vi "Main.vi"(8 "error in (no error)":errorcluster, 11 "App in":refnum<class "App.lvclass">) -> (0 "error out":errorcluster)   [LabVIEW 2020, in "Volatus.lvlib"]
uses:
  Volatus.lvlib
  App/App.lvclass
  VolatusCoreTask/VolatusCoreTask.lvclass
  C:/Program Files (x86)/National Instruments/LabVIEW 2020/vi.lib/ActorFramework/Actor/Actor.lvclass
  <vilib>/ActorFramework/Actor/Actor.lvclass
  lv-promises/Promises/Promise/Promise.lvclass
  lv-promises/Promises/Error Result/Error Result.lvclass
  lv-promises/Promises/Future/Future.lvclass
  C:/dev/lv20CE/relink/lv-promises/Promises/Value/Value.lvclass
  C:/dev/lv20CE/relink/lv-promises/Promises/Error Result/Error Result.lvclass
  C:/dev/lv20CE/relink/lv-volatus/Volatus/Task/Task.lvclass
  C:/dev/lv20CE/relink/lv-volatus/Volatus/APIRegistrationHandler/APIRegistrationHandler.lvclass
  C:/dev/lv20CE/relink/lv-volatus/Volatus/TaskStateHandler/TaskStateHandler.lvclass
  C:/dev/lv20CE/relink/lv-volatus/Volatus/VectoMessageHandler/VectoMessageHandler.lvclass
  C:/dev/lv20CE/relink/lv-volatus/Volatus/VolatusCoreTask/VolatusCoreTask.lvclass
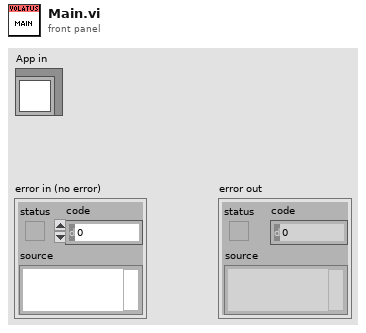
[diagram p1: front panel]
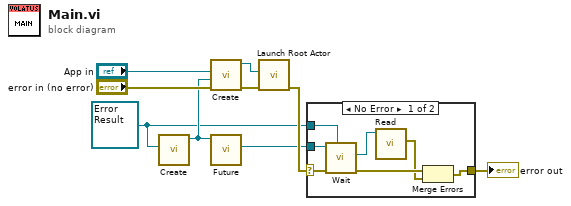
[diagram p0: block diagram]
diagram:
  w2 = refnum<class "Error Result.lvclass"> refnum ("Futures:Error Result.lvclass")
  n1 = call "Create.vi"("Result Type"=w2) -> ("Promise"=w4:refnum<class "Promise.lvclass">)  [unwired: 9 in, 1 out]
  n2 = call "Create.vi"("error in (no error)"="error in (no error)", "Promise"=w4, "App"="App in") -> ("error out"=w6:errorcluster, "VolatusCore out"=w5:refnum<class "VolatusCoreTask.lvclass">)  [unwired: 7 in]
  n3 = call "Future.vi"("Promise in"=w4) -> ("Future"=w3:refnum<class "Future.lvclass">)  [unwired: 9 in, 1 out]
  n4 = call <vilib>:"Launch Root Actor.vi"("error in (no error)"=w6, "Actor"=w5) -> ("error out"=w9:errorcluster)  [unwired: 8 in, 1 out]
  n5 = case shown="No Error" w9 {
    selector: w9 -> [w15 w17]
    tunnel: w3 -> [w16 _]
    tunnel: w2 -> [w14 _]
    tunnel: [w10 w17] -> w1
    frame No Error {
      n6 = call "Wait.vi"("Result Type"=w14, "error in (no error)"=w15, "Future in"=w16) -> ("error out"=w12:errorcluster, "Result"=w13:refnum<class "Error Result.lvclass">)  [unwired: 7 in]
      n7 = call "Read.vi"("Error Result in"=w13) -> ("Error"=w11:errorcluster)  [unwired: 10 in]
      n8 = Merge Errors(w12, w11) -> (w10:errorcluster)
    }
    frame Error {
    }
  }
  "error out" <- w1
